vi "tlacitkoNahoru.vi"(11 "NXT/EV3":T1) -> (0 "Boolean":bool, 3 "NXT/EV3 2":T1)   [LabVIEW 2013]
uses:
  <vilib>/NXT/Subs/LVHSConnector.ctl
  <vilib>/NXT/LegoClasses/BrickReference/BrickReference.lvclass
  <vilib>/NXT/Block Support/NXT_ButtonSelector.ctl
  <vilib>/NXT/Dual Mode Library/Advanced/NXTFlag_Get_Integer.vi
  <vilib>/NXT/Dual Mode Library/Sensors/readNXTButton.vi
  <vilib>/NXT/Dual Mode Library/Sensors/EV3_Infrared_Remote.vi
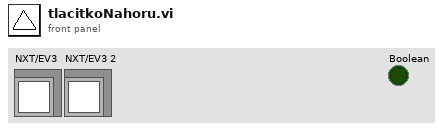
[diagram p1: front panel]
types:
  T1 = typedef "LVHSConnector.ctl" = refnum<class "BrickReference.lvclass">
  T2 = typedef "NXT_ButtonSelector.ctl" = u16
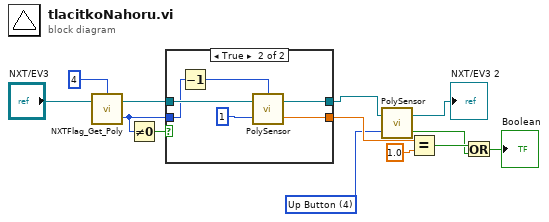
[diagram p0: block diagram]
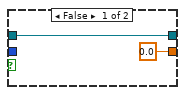
[diagram p2: hidden frame]
diagram:
  w11 = T2 4 items=["Enter button"=3, "Left button"=2, "Right button"=1, "Up Button"=4, "Down Button"=5] ("Button (Enter button)")
  n1 = call-poly <vilib>:"NXTFlag_Get_Poly.vi"("NXT/EV3"="NXT/EV3", "NXT/EV3 Flag Number"=4) -> ("Flag Value"=w3:i32, "NXT/EV3"=w7:T1)  [unwired: 1 in]
  n2 = Not Equal To 0?(x=w3) -> (x != 0?=w6:bool)
  n3 = case shown="True" w6 {
    tunnel: [sgl 0.0 ("Button Detected") w21] -> w13
    tunnel: w7 -> [w14 w19]
    tunnel: [w14 w18] -> w2
    tunnel: w3 -> [_ w16]
    frame False {
    }
    frame True {
      n4 = Decrement(x=w16) -> (x-1=w17:i32)
      n5 = call-poly <vilib>:"PolySensor.vi"("Channel"=u8 1, "NXT/EV3"=w19, "Port (Port 1)"=w17) -> ("Button Detected"=w21:sgl, "NXT/EV3"=w18:T1)
    }
  }
  n6 = call-poly <vilib>:"PolySensor.vi"("Button (Enter button)"=w11, "NXT/EV3"=w2) -> ("Yes/No"=w8:bool, "NXT/EV3"=→"NXT/EV3 2":T1)  [unwired: 1 in]
  n7 = Equal?(x=w13, y=sgl 1.0) -> (x = y?=w9:bool)
  n8 = Or(x=w9, y=w8) -> (x .or. y?=→"Boolean":bool)
